vi "ReturnValues.vi"(6 "error in":errorcluster, 9 "TopLevelDiagram in":refnum<class "TopLevelDiagram.lvclass">) -> (0 "error out":errorcluster, 3 "TopLevelDiagram out":refnum<class "TopLevelDiagram.lvclass">, 4 "inputs":string[](array[string]), 5 "return":string)   [LabVIEW 2014, in "Raspberry Pi Compatible Compiler for LabVIEW.lvlib" / "TopLevelDiagram.lvclass"]
uses:
  TopLevelDiagram.lvclass
  Python/Parsing/ListTypesTD.ctl
  Terminal/Terminal.lvclass
  Python/Parsing/Python Functions.lvlib
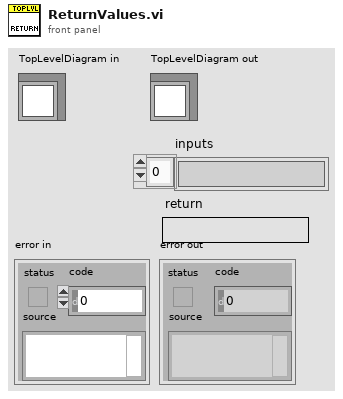
[diagram p1: front panel]
types:
  T1 = typedef "Raspberry Pi Compatible Compiler for LabVIEW.lvlib/Python Functions.lvlib/ListTypesTD.ctl" = enum16{"list", "tuple", "parameter list", "output list", "return values"}
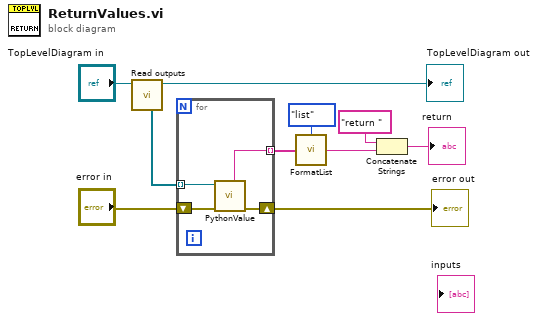
[diagram p0: block diagram]
diagram:
  n1 = call-dynamic "Read outputs.vi"("Diagram in"="TopLevelDiagram in") -> ("Diagram out"=→"TopLevelDiagram out":refnum<class "TopLevelDiagram.lvclass">, "outputs"=w7:refnum<class "Terminal.lvclass">[])  [unwired: 7 in]
  n2 = for {
    tunnel: w7 -> [w13] mode=indexing
    tunnel: [w12] -> w6 mode=indexing
    shift-right: [w11] -> w1
    shift-left: "error in" -> [w14]
    n3 = call-dynamic "PythonValue.vi"("error in"=w14, "GObject in"=w13) -> ("error out"=w11:errorcluster, "value"=w12:string)  [unwired: 7 in, 1 out]
  }
  "error out" <- w1
  n4 = call "FormatList.vi"("values"=w6, "type"=ListTypesTD."list") -> ("python object"=w3:string)
  n5 = Concatenate Strings("return " ("string"), w3) -> (→"return":string)
